vi "Init.vi"(8 "error in (no error)":errorcluster) -> (0 "error out":errorcluster, 3 "SequenceCountService out":refnum<class "SequenceCountService.lvclass">)   [LabVIEW 2020, in "Vecto.lvlib" / "SequenceCountService.lvclass"]
uses:
  SequenceCountService.lvclass
  SequenceCountService.lvclass/SequenceCountService.ctl
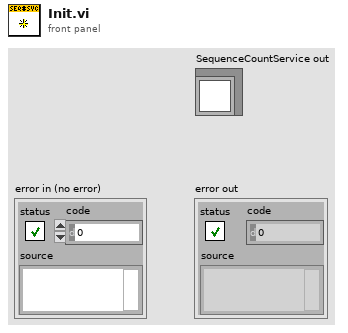
[diagram p1: front panel]
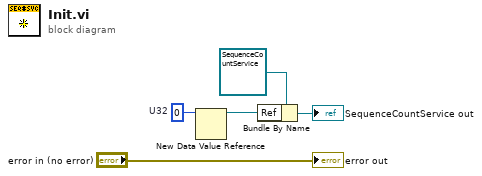
[diagram p0: block diagram]
diagram:
  w5 = u32 0  # U32
  n1 = New Data Value Reference(data value=w5) -> (data value reference=w3:refnum<data-value>)  [unwired: 1 in, 1 out]
  n2 = Bundle By Name(cluster=refnum<class "SequenceCountService.lvclass"> refnum ("SequenceCountService in"), "Ref"=w3) -> (→"SequenceCountService out":refnum<class "SequenceCountService.lvclass">)
  "error out" <- "error in (no error)"
